vi "PPL Load Help File_stub.vi"(8 "error in (no error)":errorcluster, 9 "HTML File to Load":string="MainPage_J1939.html", 10 "Main CHM File":string="J1939.chm", 11 "Browser":refnum<k7>(container)) -> (0 "error out":errorcluster)   [LabVIEW 2019]
doc: "Loads the specified HTML page from the CHM into the browser"
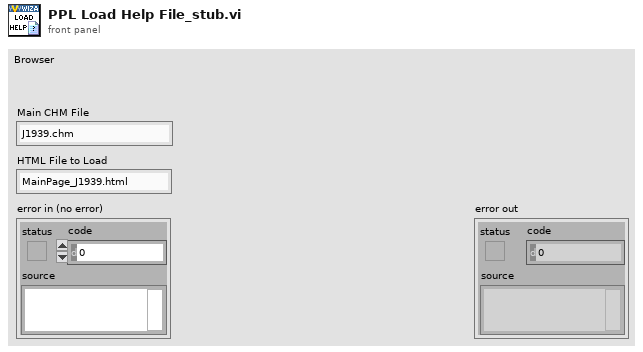
[diagram p1: front panel]
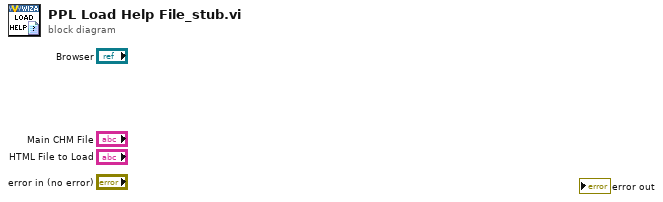
[diagram p0: block diagram]
diagram:
